vi "KHE - Save Settings.vi"(8 "error in (no error)":errorcluster, 10 "Instrument Locations":T7, 11 "Instruments":T6={"Magnet"=enum."Manual", "Ammeter"=enum."648X", "Current Source"=enum."622X", "Switch"=enum."3706A", "Voltmeter"=enum."2182A"}) -> (0 "error out":errorcluster)   [LabVIEW 2016]
uses:
  Hall Effect Library/Public/Controls/Magnets.ctl
  Hall Effect Library/Public/Controls/Ammeters.ctl
  Hall Effect Library/Public/Controls/I-Sources.ctl
  Hall Effect Library/Public/Controls/Switches.ctl
  Hall Effect Library/Public/Controls/Voltmeters.ctl
  Hall Effect Library/Hall Effect Library.lvlib
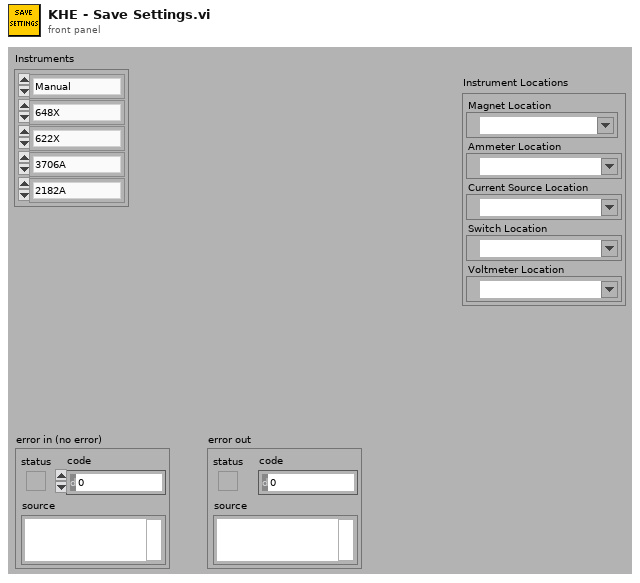
[diagram p1: front panel]
types:
  T1 = typedef "Hall Effect Library.lvlib/Magnets.ctl" = enum16{"Manual"}
  T2 = typedef "Hall Effect Library.lvlib/Ammeters.ctl" = enum16{"None", "648X"}
  T3 = typedef "Hall Effect Library.lvlib/I-Sources.ctl" = enum16{"622X", "26XX"}
  T4 = typedef "Hall Effect Library.lvlib/Switches.ctl" = enum16{"3706A"}
  T5 = typedef "Hall Effect Library.lvlib/Voltmeters.ctl" = enum16{"2000", "2182A", "3706A"}
  T6 = cluster{"Magnet":T1, "Ammeter":T2, "Current Source":T3, "Switch":T4, "Voltmeter":T5}
  T7 = cluster{"Magnet Location":refnum<visa-resource-name>, "Ammeter Location":refnum<visa-resource-name>, "Current Source Location":refnum<visa-resource-name>, "Switch Location":refnum<visa-resource-name>, "Voltmeter Location":refnum<visa-resource-name>}
  T8 = cluster{"Instruments":cluster{"Magnet":T1, "Ammeter":T2, "Current Source":T3, "Switch":T4, "Voltmeter":T5}, "Instrument Locations":cluster{"Magnet Location":refnum<visa-resource-name>, "Ammeter Location":refnum<visa-resource-name>, "Current Source Location":refnum<visa-resource-name>, "Switch Location":refnum<visa-resource-name>, "Voltmeter Location":refnum<visa-resource-name>}}
  T9 = enum16{"open", "replace", "create", "open or create", "replace or create", "replace or create with confirmation"}
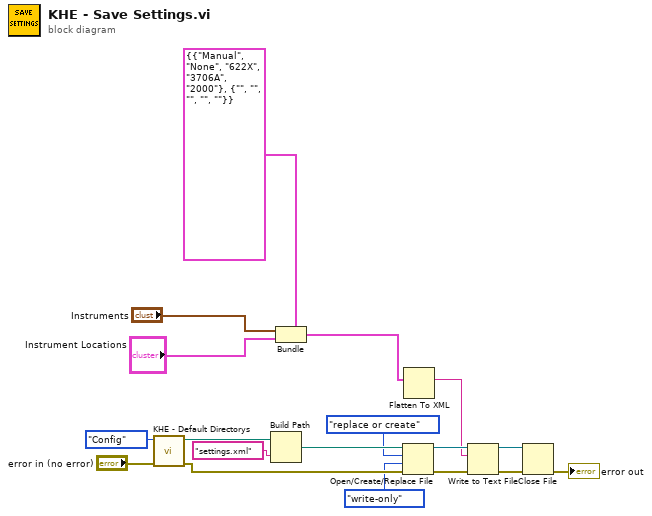
[diagram p0: block diagram]
diagram:
  n1 = call "KHE - Default Directorys.vi"("error in (no error)"="error in (no error)", "Directory"=enum16{"Root", "Config", "Results"}."Config") -> ("error out"=w13:errorcluster, "Path Out"=w15:path)  [unwired: 8 out]
  n2 = Build Path(base path=w15, name or relative path="settings.xml") -> (appended path=w14:path)
  n3 = Bundle(cluster=T8 {"Instruments"={"Magnet"=enum."Manual", "Ammeter"=enum."None", "Current Source"=enum."622X", "Switch"=enum."3706A", "Voltmeter"=enum."2000"}, "Instrument Locations"={"Magnet Location"="", "Ammeter Location"="", "Current Source Location"="", "Switch Location"="", "Voltmeter Location"=""}} ("output cluster"), "Instruments"="Instruments", "Instrument Locations"="Instrument Locations") -> (w2:T8)
  n4 = Open/Create/Replace File(file path (use dialog)=w14, error in=w13, operation (0:open)=T9."replace or create", access (0:read/write)=enum16{"read/write", "read-only", "write-only"}."write-only") -> (refnum out=w9:refnum<file>, error out=w10:errorcluster)  [unwired: 3 out]
  n5 = Flatten To XML(anything=w2) -> (xml string=w8:string)
  n6 = Write to Text File(file (use dialog)=w9, text=w8, error in=w10) -> (refnum out=w7:refnum<file>, error out=w6:errorcluster)  [unwired: 2 out]
  n7 = Close File(refnum=w7, error in=w6) -> (error out=→"error out":errorcluster)  [unwired: 1 out]
